vi "DefaultFromIni.vi"(8 "error in (no error)":errorcluster, 11 "NhRegenGridSim":refnum<class "NHRGridSim.lvclass">) -> (0 "error out":errorcluster, 3 "NhRegenGridSim":refnum<class "NHRGridSim.lvclass">)   [LabVIEW 2018, in "AcPwrPlugins.lvlib" / "NHRGridSim.lvclass"]
doc: "This VI reads the properties from the INI file and puts them into the LabVIEW class for further use."
uses:
  NHRGridSim.lvclass
  C:/Program Files (x86)/National Instruments/LabVIEW 2018/user.lib/NIST/BaseClasses/BasePlugin_class/BasePlugin.lvclass
  Measurements.ctl
  TypeDefs/DeviceSettings.ctl
  <userlib>/NIST/BaseClasses/BasePlugin_class/BasePlugin.lvclass/BasePlugin.ctl
  <userlib>/NIST/BaseClasses/BasePlugin_class/Accessors/Read PluginIniFilePath.vi
  AcPwrBaseClass/AcPwrBase.lvclass
  <vilib>/Utility/config.llb/NI_LVConfig.lvlib
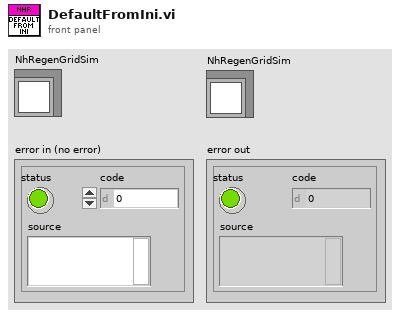
[diagram p1: front panel]
types:
  T1 = typedef "AcPwrPlugins.lvlib/NHRGridSim.lvclass/DeviceSettings.ctl" = cluster{"SlewRates":cluster{"Islew":dbl, "Vslew":dbl, "Pslew":dbl, "FreqSlew":dbl, "AngleABSlew":dbl, "AngleACSlew":dbl}, "Phases":cluster{"Pout (W)":dbl, "Iout (A)":dbl, "PhaseAngle":dbl, "Vout (V)":dbl, "Phase Name":string}[], "Measurement":cluster{"ApertureLength (s)":dbl, "NumberOfSamples":u32}, "Ranges":cluster{"Irange (A)":dbl, "Vrange (V)":dbl}, "Mode":enum8{"One 3-Phase AC", "One AC", "One DC", "Three AC", "Three DC", "One 2-Phase AC and One AC", "One 2-Phase AC and One DC", "Two AC", "One AC and One DC", "Two AC and One DC", "One AC and Two DC", "One DC and One AC", "Two DC"}, "PowerMax":u16, "TransformerRatio":dbl, "Waveshape":dbl[], "Handle":string, "FreqOut (Hz)":dbl, "Connected":bool, "Safety Limits":cluster{"Minimum Voltage (V)":dbl, "Minimum Voltage Time (s)":dbl, "Maximum Voltage (V)":dbl, "Maximum Voltage Time (s)":dbl, "Maximum Source Amps (A)":dbl, "Maximum Source Amps Time (s)":dbl, "Maximum Sink Amps (A)":dbl, "Maximum Sink Amps Time (s)":dbl, "Maximum Source Power (W)":dbl, "Maximum Source Power Time (s)":dbl, "Maximum Sink Power (W)":dbl, "Maximum Sink Power Time (s)":dbl, "Peak Voltage (V)":dbl, "Peak Voltage Enable":bool, "Peak Amps (A)":dbl, "Peak Amps Enable":bool}, "btnIdQuery":bool, "btnReset":bool, "Initialize Timeout (10000 ms)":u32}[]
  T2 = typedef "AcPwrPlugins.lvlib/NHRGridSim.lvclass/Measurements.ctl" = cluster{"Handle":string, "Name":string, "Enabled ":bool, "Measurement Value":dbl, "Measurement Type ":enum16{"Average Current", "Max Current", "Min Current", "Average Voltage", "Max Voltage", "Min Voltage", "Average True Power", "Max True Power", "Min True Power", "Average Apparent Power", "Max Apparent Power", "Min Apparent Power", "Power Factor", "Crest Factor"}, "Phase ":i32, "btnMeasFetch":bool}[]
  T3 = typedef "NI_LVConfig.lvlib/Config Data RefNum.ctl" = refnum<k1>
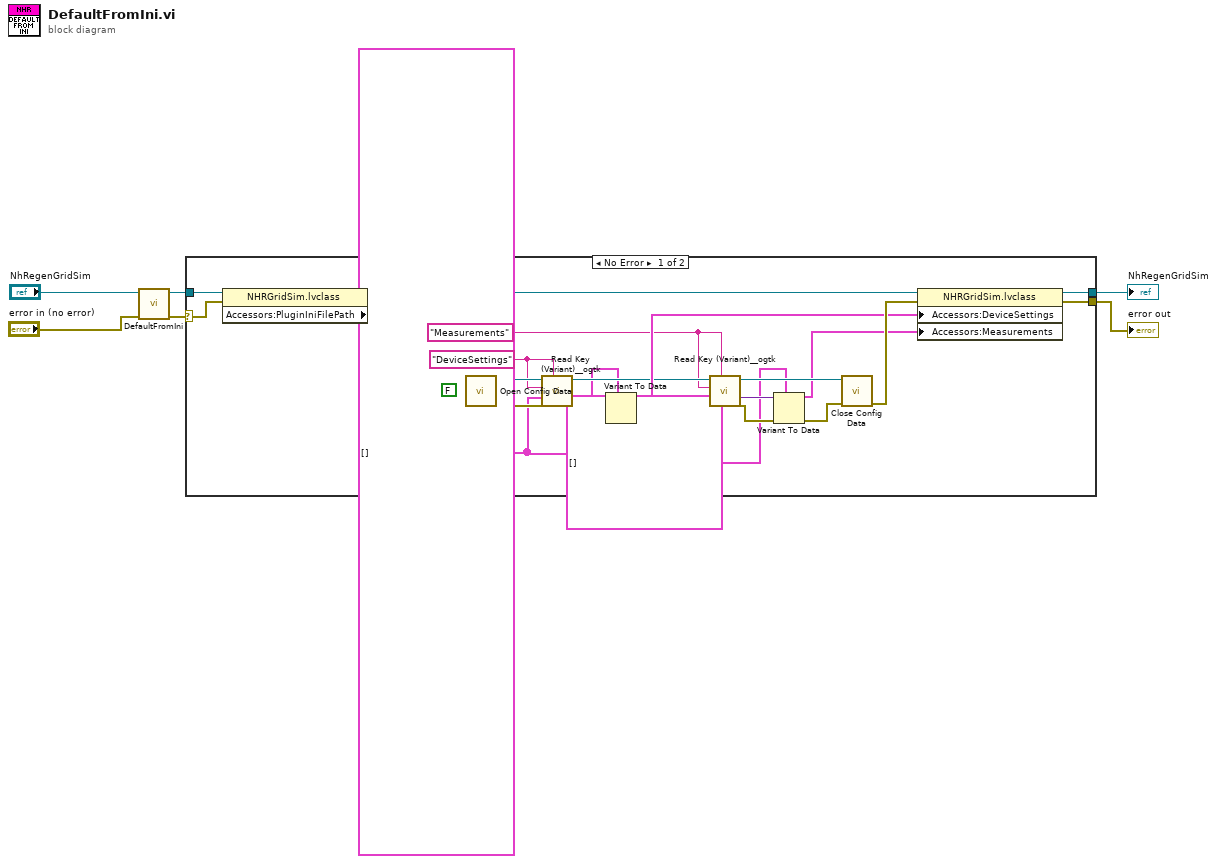
[diagram p0: block diagram]
diagram:
  n1 = call-parent "DefaultFromIni.vi"("error in (no error)"="error in (no error)", "AcPwrBase"="NhRegenGridSim") -> ("error out"=w1:errorcluster, "AcPwrBase"=w4:refnum<class "NHRGridSim.lvclass">)  [unwired: 8 in]
  n2 = case shown="No Error" w1 {
    selector: w1 -> [w21 w32]
    tunnel: w4 -> [w31 w33]
    tunnel: [w23 w33] -> w6
    tunnel: [w19 w32] -> w5
    frame No Error {
      w7 = T1 [] ("DeviceSettings")
      w8 = T2 [] ("Measurements")
      w10 = "Measurements" ("section")
      w22 = "DeviceSettings" ("section")
      n3 = property class="NHRGridSim.lvclass"(reference=w31, error in=w21) -> (reference out=w24:refnum<class "NHRGridSim.lvclass">, error out=w20:errorcluster, "Accessors:PluginIniFilePath"=w30:path)
      n4 = call <vilib>:"Open Config Data.vi"("error in (no error)"=w20, "create file if necessary (T)"=FALSE, "configuration file path"=w30) -> ("error out"=w27:errorcluster, "refnum"=w28:T3)  [unwired: 6 in, 1 out]
      n5 = call <userlib>:"Read Key (Variant)__ogtk.vi"("section"=w22, "error in (no error)"=w27, "type"=w7, "key (optional)"=w22, "refnum"=w28) -> ("error out"=w25:errorcluster, "key-value"=w26:variant, "refnum out"=w14:T3)  [unwired: 3 in, 1 out]
      n6 = Variant To Data(error in=w25, type=w7, Variant=w26) -> (data=w17:T1, error out=w11:errorcluster)
      n7 = call <userlib>:"Read Key (Variant)__ogtk.vi"("section"=w10, "error in (no error)"=w11, "type"=w8, "key (optional)"=w10, "refnum"=w14) -> ("error out"=w16:errorcluster, "key-value"=w15:variant, "refnum out"=w13:T3)  [unwired: 3 in, 1 out]
      n8 = Variant To Data(error in=w16, type=w8, Variant=w15) -> (data=w9:T2, error out=w12:errorcluster)
      n9 = call <vilib>:"Close Config Data.vi"("error in (no error)"=w12, "refnum"=w13) -> ("error out"=w18:errorcluster)  [unwired: 8 in, 1 out]
      n10 = property class="NHRGridSim.lvclass"(reference=w24, error in=w18, "Accessors:DeviceSettings"=w17, "Accessors:Measurements"=w9) -> (reference out=w23:refnum<class "NHRGridSim.lvclass">, error out=w19:errorcluster)
    }
    frame Error {
    }
  }
  "error out" <- w5
  "NhRegenGridSim" <- w6
